vi "2DRasterScanWithScopeCommAndSafeRetract.vi"() -> ()   [LabVIEW 2015]
panel:
  in  "Swap X and Z?":bool
  out "Progress":u8(slide)=96 scale=0.0..100.0
  out "Z-error":errorcluster
  out "X-error":errorcluster
  in  "Z safe retract":sgl=25.0
  in  "MG17Motor Z axis":refnum<k7>(container)
  in  "Home Z?":bool
  in  "Z-Axis Serial":i32=27001113
  in  "Safe retract?":bool=TRUE
  in  "X safe retract":sgl=100.0
  in  "Y safe retract":sgl=25.0
  out "Y error":errorcluster
  in  "Base filename":string="TDS" caption="Filename"
  in  "Save Each Point":bool=TRUE
  in  "X-Axis Serial":i32=45869591
  in  "Y-Axis Serial":i32=27501169
  out "Number of movements for Y stage":sgl=49.0
  in  "Distance from center X axis (mm)":dbl=2.0 step=0.001
  in  "Movement Step Size X axis (mm)":sgl=0.25 step=0.001
  in  "Channel Select":T1(ring)=enum."Channel 1"
  in  "Selected Directory":path=path "C:/Users/admin.WIN10DC20170225/Documents/Hydrophone Data/TDS Scans/TDS 04_04_18 BarePZT-20ms-XY"
  in  "Stage Max Velocity (mm/s)":sgl=1.5
  in  "Stage Acceleration (mm/s²)":sgl=1.0
  in  "Stage Minimum Velocity (mm/s)":sgl
  in  "Center point Y axis (mm)":dbl=20.0 step=0.001 format="%#_13g"
  in  "Center point X axis (mm)":dbl=63.5 step=0.001 format="%#_13g"
  out "Number of movements for X stage":sgl=49.0
  in  "Distance from center Y axis (mm)":dbl=2.0 step=0.001
  in  "MG17Motor X axis":refnum<k7>(container)
  in  "Home stages\nbefore scanning":bool caption="Do this each time LabVIEW  is opened, controllers are unplugged, or stages are disconnected."
  in  "error in (no error)":errorcluster
  in  "MG17Motor Y axis":refnum<k7>(container)
  out "Current position in line":i32=49
  out "Current line number":i32=49
  in  "Movement Step Size Y axis (mm)":sgl=0.25 step=0.001
  # "BEFORE STARTING SCAN ENSURE THAT X-Z AXIS SWAPPING AND SAFE RETRACT VALUES ARE PROPERLY SET"
  # "Use safe retract to pull hydrophone out of water when scan is finished. Normal retraction order is Y -> X -> Z"
  # "When X and Z are swapped,\nretraction order is Y -> Z -> X"
  # "For Y-Z scans- turn this on and then treat X values as Z."
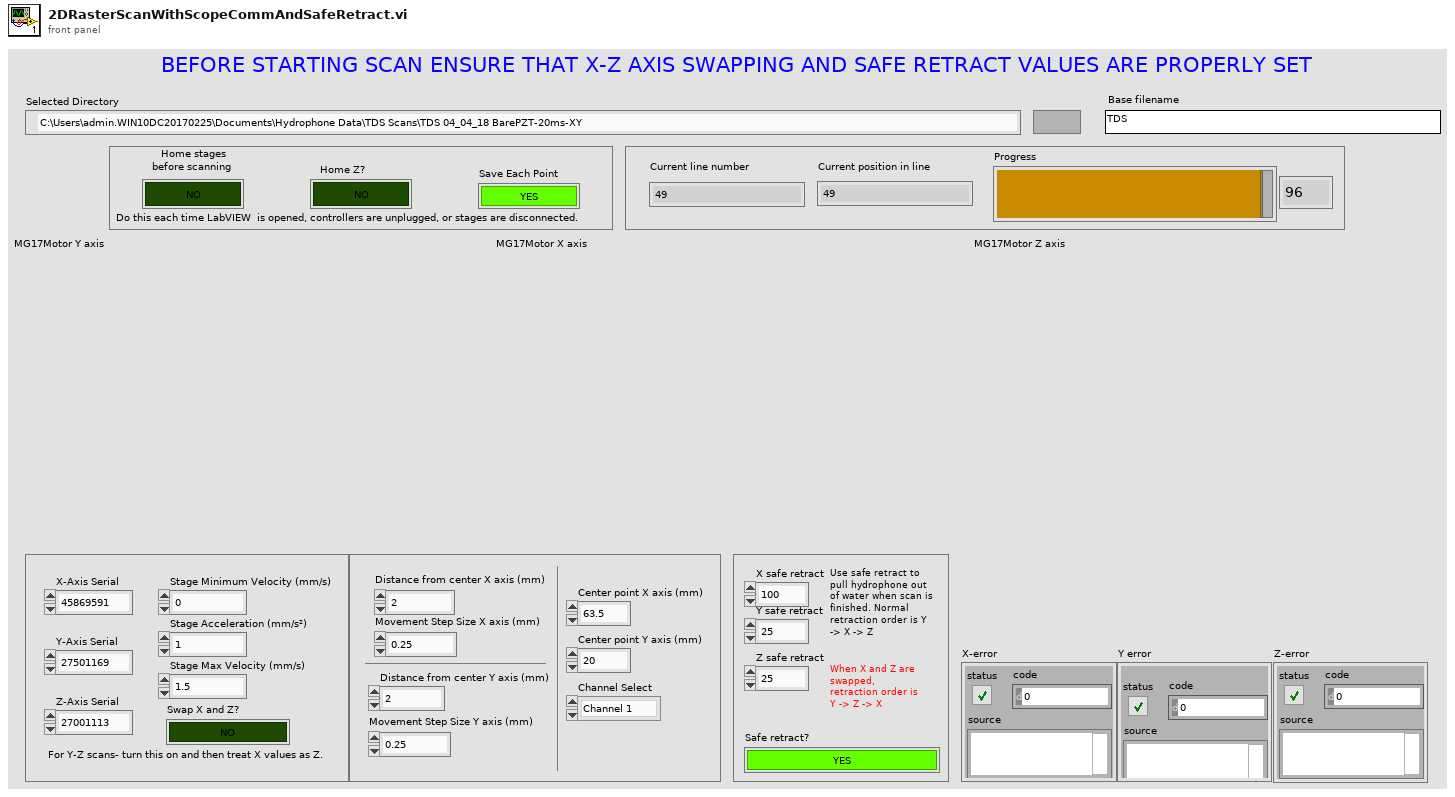
[diagram p1: front panel]
types:
  T1 = enum16{"Trace D", "Trace C", "Trace B", "Trace A", "Channel 4", "Channel 3", "Channel 2", "Channel 1"}
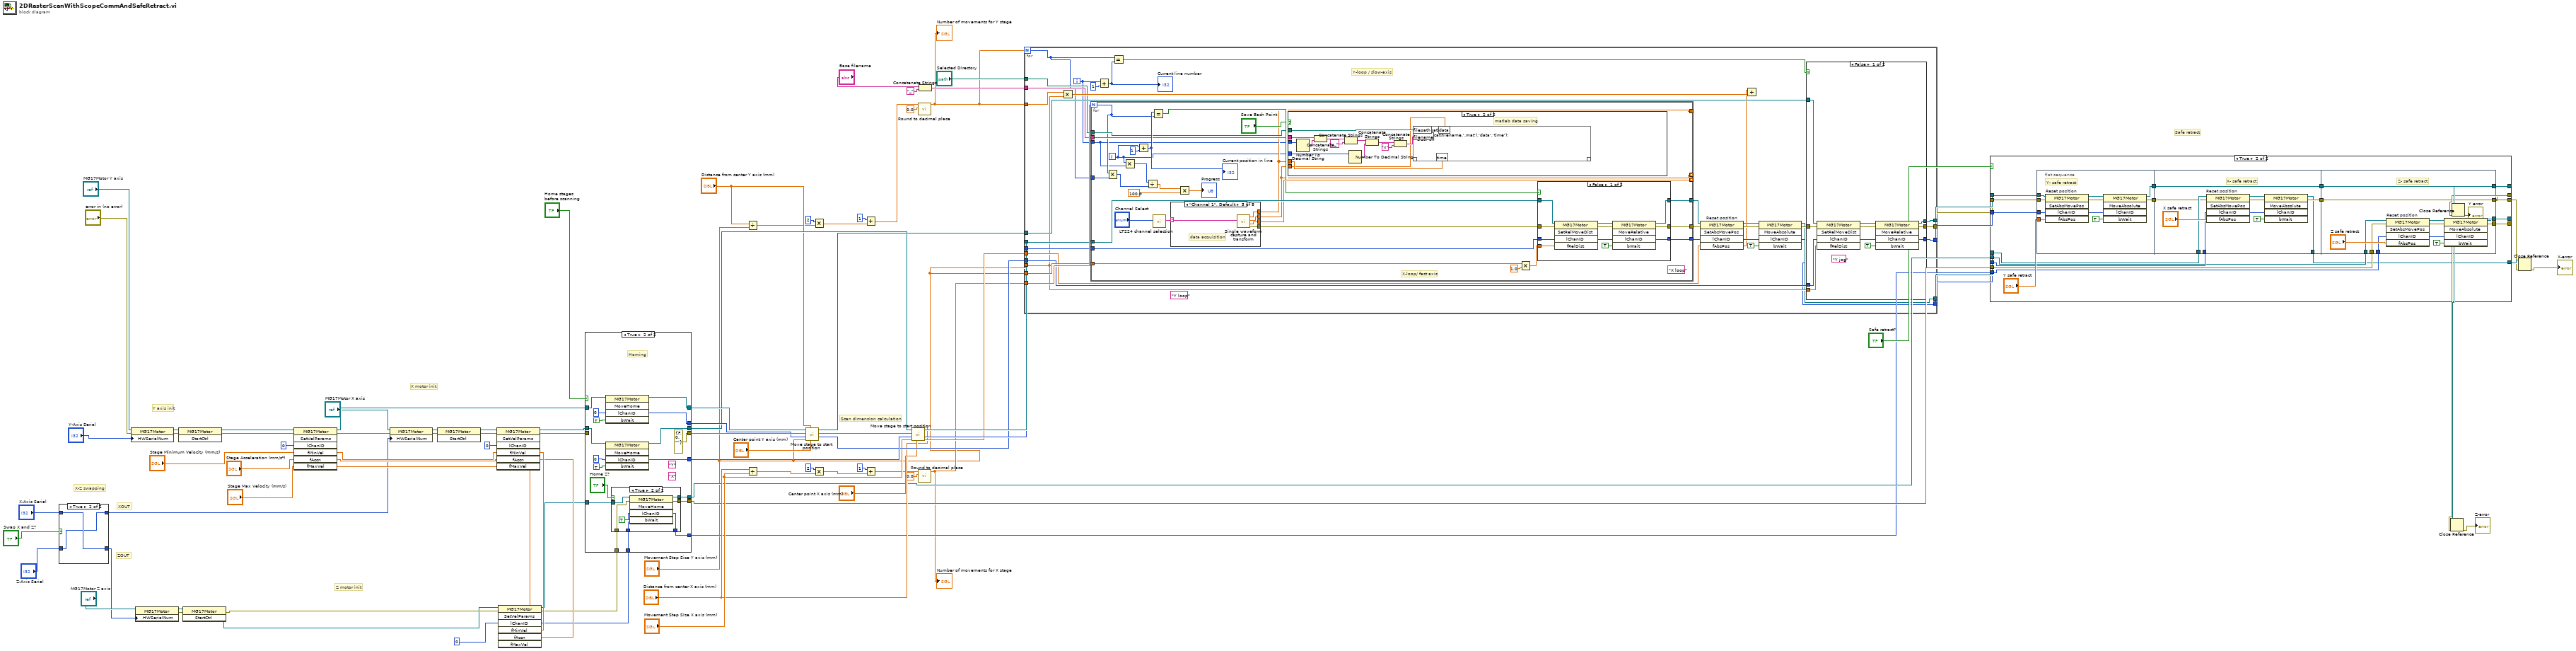
[diagram p0: block diagram]
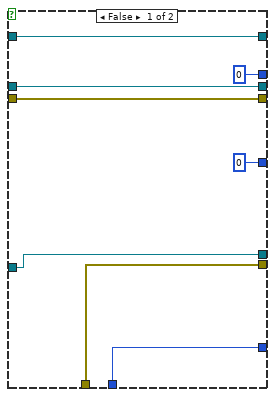
[diagram p4: hidden frame]
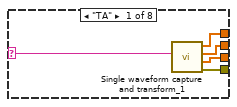
[diagram p9: hidden frame]
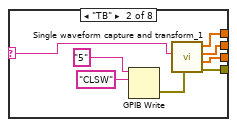
[diagram p10: hidden frame]
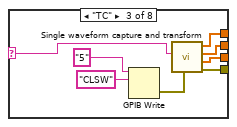
[diagram p11: hidden frame]
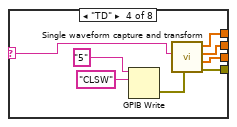
[diagram p12: hidden frame]
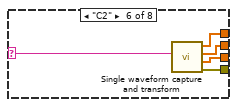
[diagram p13: hidden frame]
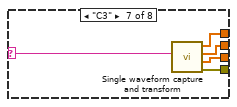
[diagram p14: hidden frame]
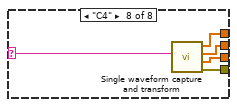
[diagram p15: hidden frame]
diagram:
  # "Scan dimension calculation"
  # "X-Z swapping"
  # "Y axis init"
  # "Z motor init"
  # "X motor init"
  # "ZOUT"
  # "XOUT"
  # "Safe retract"
  n1 = case shown="True" "Swap X and Z?" {
    tunnel: "X-Axis Serial" -> [w97 w99]
    tunnel: [w97 w98] -> w6
    tunnel: "Z-Axis Serial" -> [w96 w98]
    tunnel: [w96 w99] -> w5
    frame False {
    }
    frame True {
    }
  }
  n2 = property on="Property Node" class="MG17Motor"(reference="MG17Motor Y axis", error in="error in (no error)", "HWSerialNum"="Y-Axis Serial") -> (reference out=w94:refnum<k7>, error out=w93:errorcluster)
  n3 = property on="Property Node" class="MG17Motor"(reference="MG17Motor Z axis", "HWSerialNum"=w5) -> (reference out=w27:refnum<k7>, error out=w28:errorcluster)  [unwired: 1 in]
  n4 = invoke class="MG17Motor" method="StartCtrl"(reference=w94, error in=w93) -> (reference out=w86:refnum<k7>, error out=w87:errorcluster)  [unwired: 1 in, 1 out]
  n5 = invoke class="MG17Motor" method="StartCtrl"(reference=w27, error in=w28) -> (reference out=w23:refnum<k7>, error out=w22:errorcluster)  [unwired: 1 in, 1 out]
  n6 = invoke class="MG17Motor" method="SetVelParams"(reference=w86, error in=w87, "lChanID"=0, "fMinVel"="Stage Minimum Velocity (mm/s)", "fAccn"="Stage Acceleration (mm/s²)", "fMaxVel"="Stage Max Velocity (mm/s)") -> (reference out=w75:refnum<k7>, error out=w76:errorcluster, "fMinVel"=w56:sgl, "fAccn"=w55:sgl, "fMaxVel"=w54:sgl)  [unwired: 1 in, 2 out]
  n7 = property on="Property Node" class="MG17Motor"(reference="MG17Motor X axis", error in=w76, "HWSerialNum"=w6) -> (reference out=w89:refnum<k7>, error out=w88:errorcluster)
  n8 = invoke class="MG17Motor" method="StartCtrl"(reference=w89, error in=w88) -> (reference out=w85:refnum<k7>, error out=w78:errorcluster)  [unwired: 1 in, 1 out]
  n9 = invoke class="MG17Motor" method="SetVelParams"(reference=w85, error in=w78, "lChanID"=0, "fMinVel"=w56, "fAccn"=w55, "fMaxVel"=w54) -> (reference out=w84:refnum<k7>, error out=w77:errorcluster, "fMinVel"=w26:sgl, "fAccn"=w25:sgl, "fMaxVel"=w24:sgl)  [unwired: 1 in, 2 out]
  n10 = invoke class="MG17Motor" method="SetVelParams"(reference=w23, error in=w22, "lChanID"=0, "fMinVel"=w26, "fAccn"=w25, "fMaxVel"=w24) -> (reference out=w20:refnum<k7>, error out=w19:errorcluster, "lChanID"=w14:i32)  [unwired: 1 in, 4 out]
  n11 = case shown="True" "Home stages\nbefore scanning" {
    tunnel: [w104 w121] -> w65
    tunnel: [w105 w120] -> w71
    tunnel: [0 ("lChanID") w119] -> w66
    tunnel: [0 ("lChanID") w118] -> w69
    tunnel: [w103 errorcluster {"status"=FALSE, "code"=0, "source"=""} ("error out")] -> w70
    tunnel: w75 -> [w105 w116]
    tunnel: w84 -> [w104 w115]
    tunnel: w77 -> [w103 _]
    tunnel: w20 -> [w102 w113]
    tunnel: w19 -> [w101 w112]
    tunnel: [w102 w111] -> w17
    tunnel: [w101 w110] -> w16
    tunnel: w14 -> [w100 w109]
    tunnel: [w100 w108] -> w13
    frame False {
    }
    frame True {
      (unwired) "X"
      (unwired) "Y"
      # "Homing"
      n12 = invoke class="MG17Motor" method="MoveHome"(reference=w116, "lChanID"=0, "bWait"=TRUE) -> (reference out=w120:refnum<k7>, "lChanID"=w118:i32)  [unwired: 2 in, 3 out]
      n13 = invoke class="MG17Motor" method="MoveHome"(reference=w115, "lChanID"=0, "bWait"=TRUE) -> (reference out=w121:refnum<k7>, "lChanID"=w119:i32)  [unwired: 2 in, 3 out]
      n14 = case shown="True" "Home Z?" {
        tunnel: w113 -> [w128 w134]
        tunnel: w112 -> [w127 w133]
        tunnel: [w128 w132] -> w111
        tunnel: [w127 w131] -> w110
        tunnel: w109 -> [w126 w130]
        tunnel: [w126 w129] -> w108
        frame False {
        }
        frame True {
          n15 = invoke class="MG17Motor" method="MoveHome"(reference=w134, error in=w133, "lChanID"=w130, "bWait"=TRUE) -> (reference out=w132:refnum<k7>, error out=w131:errorcluster, "lChanID"=w129:i32)  [unwired: 1 in, 2 out]
        }
      }
    }
  }
  n16 = Divide(x="Distance from center Y axis (mm)", y="Movement Step Size Y axis (mm)") -> (x/y=w59:dbl)
  n17 = Divide(x="Distance from center X axis (mm)", y="Movement Step Size X axis (mm)") -> (x/y=w51:dbl)
  n18 = call "Move stage to start position.vi"("Center point of axis (mm)"="Center point Y axis (mm)", "Distance from center (mm)"="Distance from center Y axis (mm)", "Movement Step Size (mm)"="Movement Step Size Y axis (mm)", "lChanID"=w69, "error in"=w70, "reference in"=w71) -> ("lChanID out"=w60:i32, "error out"=w67:errorcluster, "reference out"=w68:refnum<k7>)  [unwired: 2 in, 1 out]
  n19 = Multiply(x=2, y=w59) -> (x*y=w73:dbl)
  n20 = Multiply(x=2, y=w51) -> (x*y=w52:dbl)
  n21 = Add(x=1, y=w73) -> (x+y=w46:dbl)
  n22 = Add(x=1, y=w52) -> (x+y=w47:dbl)
  n23 = call "Move stage to start position.vi"("Center point of axis (mm)"="Center point X axis (mm)", "Distance from center (mm)"="Distance from center X axis (mm)", "Movement Step Size (mm)"="Movement Step Size X axis (mm)", "lChanID"=w66, "error in"=w67, "reference in"=w65) -> ("Start position out"=w61:sgl, "lChanID out"=w62:i32, "reference out"=w63:refnum<k7>)  [unwired: 2 in, 1 out]
  n24 = call "Round to decimal place.vi"("Power of ten"=0.0, "Number to round"=w46) -> ("Rounded number"=w1:dbl)  [unwired: 8 in, 1 out]
  "Number of movements for Y stage" <- w1
  n25 = call "Round to decimal place.vi"("Power of ten"=0.0, "Number to round"=w47) -> ("Rounded number"=w4:dbl)  [unwired: 8 in, 1 out]
  "Number of movements for X stage" <- w4
  n26 = Concatenate Strings("Base filename", "_" ("string")) -> (w40:string)
  n27 = for {
    N: w1 -> [w137]
    tunnel: "Movement Step Size Y axis (mm)" -> [w161]
    tunnel: w4 -> [w166]
    tunnel: [w156] -> w37
    tunnel: [w155] -> w12
    tunnel: "Movement Step Size Y axis (mm)" -> [w148]
    tunnel: w68 -> [w154]
    tunnel: w63 -> [w153]
    tunnel: w62 -> [w152]
    tunnel: w61 -> [w151]
    tunnel: w60 -> [w150]
    tunnel: w1 -> [w147]
    tunnel: w40 -> [w143]
    tunnel: "Selected Directory" -> [w142]
    tunnel: [w140] -> w35
    tunnel: [w139] -> w36
    tunnel: [w138] -> w34
    i -> [w141]
    (unwired) "Y loop"
    # "Y-loop / slow-axis"
    n28 = Multiply(x=w147, y=w148) -> (x*y=w149:dbl)
    n29 = for {
      N: w166 -> [w188]
      tunnel: w161 -> [w201]
      tunnel: [w190] -> _
      tunnel: [w205] -> w144
      tunnel: [w206] -> w159
      tunnel: [w204] -> w158
      tunnel: [w198] -> _ mode=indexing
      tunnel: w153 -> [w202]
      tunnel: w152 -> [w203]
      tunnel: [w193] -> _ mode=indexing
      tunnel: w143 -> [w194]
      tunnel: w142 -> [w192]
      tunnel: w141 -> [w187]
      tunnel: w137 -> [w189]
      i -> [w184]
      (unwired) "X loop"
      # "X-loop/ fast axis"
      n30 = Multiply(x=w188, y=w189) -> (x*y=w181:i32)
      n31 = Multiply(x=w184, y=w187) -> (x*y=w182:i32)
      n32 = Add(x=w184, y=1) -> (x+y=w195:i32)
      "Current position in line" <- w195
      n33 = Divide(x=w182, y=w181) -> (x/y=w183:dbl)
      n34 = Equal?(x=w195, y=w188) -> (x = y?=w196:bool)
      n35 = call "LT224 channel selection.vi"("Channel Select"="Channel Select") -> ("Selected channel"=w199:string)  [unwired: 10 in]
      n36 = case shown="\"Channel 1\", Default" w199 {
        selector: w199 -> [w239 w244 w252 w260 w268 w273 w278 w283]
        tunnel: [w242 w250 w258 w266 w271 w276 w281 w286] -> w197
        tunnel: [w241 w249 w257 w265 w270 w275 w280 w285] -> w198
        tunnel: [w240 w248 w256 w264 w269 w274 w279 w284] -> w190
        tunnel: [w238 w243 w251 w259 w267 w272 w277 w282] -> w193
        frame "TA" {
          n37 = call "Single waveform capture and transform_1.vi"("channel name (\"\")"=w239) -> ("error out"=w242:errorcluster, "Transformed waveform vector"=w241:dbl[], "waveform vector"=w238:dbl[], "Time vector"=w240:dbl[])  [unwired: 7 in]
        }
        frame "TB" {
          n38 = GPIB Write(0:"5" ("address string"), 1:"CLSW" ("data")) -> (6:w246:errorcluster)  [unwired: 3 in, 1 out]
          n39 = call "Single waveform capture and transform_1.vi"("error in"=w246, "channel name (\"\")"=w244) -> ("error out"=w250:errorcluster, "Transformed waveform vector"=w249:dbl[], "waveform vector"=w243:dbl[], "Time vector"=w248:dbl[])  [unwired: 6 in]
        }
        frame "TC" {
          n40 = GPIB Write(0:"5" ("address string"), 1:"CLSW" ("data")) -> (6:w254:errorcluster)  [unwired: 3 in, 1 out]
          n41 = call "Single waveform capture and transform.vi"("error in"=w254, "channel name (\"\")"=w252) -> ("error out"=w258:errorcluster, "Transformed waveform vector"=w257:dbl[], "waveform vector"=w251:dbl[], "Time vector"=w256:dbl[])  [unwired: 6 in]
        }
        frame "TD" {
          n42 = GPIB Write(0:"5" ("address string"), 1:"CLSW" ("data")) -> (6:w262:errorcluster)  [unwired: 3 in, 1 out]
          n43 = call "Single waveform capture and transform.vi"("error in"=w262, "channel name (\"\")"=w260) -> ("error out"=w266:errorcluster, "Transformed waveform vector"=w265:dbl[], "waveform vector"=w259:dbl[], "Time vector"=w264:dbl[])  [unwired: 6 in]
        }
        frame "Channel 1", Default {
          # "data acquisition"
          n44 = call "Single waveform capture and transform.vi"("channel name (\"\")"=w268) -> ("error out"=w271:errorcluster, "Transformed waveform vector"=w270:dbl[], "waveform vector"=w267:dbl[], "Time vector"=w269:dbl[])  [unwired: 7 in]
        }
        frame "C2" {
          n45 = call "Single waveform capture and transform.vi"("channel name (\"\")"=w273) -> ("error out"=w276:errorcluster, "Transformed waveform vector"=w275:dbl[], "waveform vector"=w272:dbl[], "Time vector"=w274:dbl[])  [unwired: 7 in]
        }
        frame "C3" {
          n46 = call "Single waveform capture and transform.vi"("channel name (\"\")"=w278) -> ("error out"=w281:errorcluster, "Transformed waveform vector"=w280:dbl[], "waveform vector"=w277:dbl[], "Time vector"=w279:dbl[])  [unwired: 7 in]
        }
        frame "C4" {
          n47 = call "Single waveform capture and transform.vi"("channel name (\"\")"=w283) -> ("error out"=w286:errorcluster, "Transformed waveform vector"=w285:dbl[], "waveform vector"=w282:dbl[], "Time vector"=w284:dbl[])  [unwired: 7 in]
        }
      }
      n48 = Multiply(x=w183, y=100.0) -> (x*y=→"Progress":dbl)
      n49 = case shown="True" "Save Each Point" {
        tunnel: w194 -> [_ w215]
        tunnel: w193 -> [_ w210]
        tunnel: w192 -> [_ w213]
        tunnel: w184 -> [_ w223]
        tunnel: w187 -> [_ w217]
        tunnel: w190 -> [_ w211]
        frame False {
        }
        frame True {
          # "matlab data saving"
          n50 = Number To Decimal String(number=w217) -> (decimal integer string=w214:string)  [unwired: 1 in]
          n51 = Concatenate Strings(w215, w214) -> (w222:string)
          n52 = Concatenate Strings(w222, "y_" ("string")) -> (w220:string)
          n53 = Number To Decimal String(number=w223) -> (decimal integer string=w216:string)  [unwired: 1 in]
          n54 = Concatenate Strings(w220, w216) -> (w218:string)
          n55 = Concatenate Strings(w218, "x" ("string")) -> (w212:string)
          n56 = script code="cd(filepath)\nsave(strcat(filename,'.mat'),'data','time');\nclear all"("filename"=w212, "filepath"=w213, "time"=w211, "data"=w210) -> ()  [unwired: 1 in, 1 out]
        }
      }
      n57 = Multiply(x=w201, y=sgl 1.0) -> (x*y=w208:sgl)
      n58 = case shown="False" w196 {
        tunnel: w208 -> [w234 _]
        tunnel: [w229 w235] -> w206
        tunnel: [w228 w237] -> w205
        tunnel: [w227 w236] -> w204
        tunnel: w203 -> [w226 w236]
        tunnel: w202 -> [w225 w235]
        tunnel: w197 -> [w224 w237]
        frame False {
          n59 = invoke class="MG17Motor" method="SetRelMoveDist"(reference=w225, error in=w224, "lChanID"=w226, "fRelDist"=w234) -> (reference out=w232:refnum<k7>, error out=w231:errorcluster, "lChanID"=w233:i32)  [unwired: 1 in, 2 out]
          n60 = invoke class="MG17Motor" method="MoveRelative"(reference=w232, error in=w231, "lChanID"=w233, "bWait"=TRUE) -> (reference out=w229:refnum<k7>, error out=w228:errorcluster, "lChanID"=w227:i32)  [unwired: 1 in, 2 out]
        }
        frame True {
        }
      }
    }
    n61 = Add(x=w141, y=1) -> (x+y=w145:i32)
    "Current line number" <- w145
    n62 = Equal?(x=w137, y=w145) -> (x = y?=w136:bool)
    n63 = invoke on="Reset position" class="MG17Motor" method="SetAbsMovePos"(reference=w159, error in=w144, "lChanID"=w158, "fAbsPos"=w151) -> (reference out=w162:refnum<k7>, error out=w164:errorcluster, "lChanID"=w163:i32, "fAbsPos"=w146:sgl)  [unwired: 1 in, 1 out]
    n64 = Add(x=w146, y=w149) -> ()  [unwired: 1 out]
    n65 = invoke class="MG17Motor" method="MoveAbsolute"(reference=w162, error in=w164, "lChanID"=w163, "bWait"=TRUE) -> (reference out=w139:refnum<k7>, error out=w157:errorcluster, "lChanID"=w138:i32)  [unwired: 1 in, 2 out]
    n66 = case shown="False" w136 {
      tunnel: w157 -> [w173 w180]
      tunnel: [w172 w178] -> w156
      tunnel: [w171 w180] -> w140
      tunnel: [w170 w179] -> w155
      tunnel: w148 -> [w169 _]
      tunnel: w154 -> [w168 w178]
      tunnel: w150 -> [w167 w179]
      frame False {
        (unwired) "Y jog"
        n67 = invoke class="MG17Motor" method="SetRelMoveDist"(reference=w168, error in=w173, "lChanID"=w167, "fRelDist"=w169) -> (reference out=w175:refnum<k7>, error out=w176:errorcluster, "lChanID"=w174:i32)  [unwired: 1 in, 2 out]
        n68 = invoke class="MG17Motor" method="MoveRelative"(reference=w175, error in=w176, "lChanID"=w174, "bWait"=TRUE) -> (reference out=w172:refnum<k7>, error out=w171:errorcluster, "lChanID"=w170:i32)  [unwired: 1 in, 2 out]
      }
      frame True {
      }
    }
  }
  n69 = case shown="True" "Safe retract?" {
    tunnel: w37 -> [w291 w309]
    tunnel: w36 -> [w290 w303]
    tunnel: w35 -> [w289 w307]
    tunnel: w34 -> [_ w301]
    tunnel: [w291 w306] -> w33
    tunnel: [w289 w292] -> w32
    tunnel: [w290 w293] -> w31
    tunnel: [w289 w292] -> w30
    tunnel: w17 -> [w288 w297]
    tunnel: w16 -> [w287 w296]
    tunnel: [w288 w298] -> w15
    tunnel: [w287 w294] -> w2
    tunnel: w13 -> [_ w295]
    tunnel: w12 -> [_ w302]
    frame False {
    }
    frame True {
      n70 = flat-sequence {
        tunnel: w309 -> [w315]
        tunnel: "Y safe retract" -> [w314]
        tunnel: w307 -> [w313]
        tunnel: [w312] -> w305
        tunnel: [w311] -> w304
        tunnel: w302 -> [w310]
        tunnel: w305 -> [w323]
        tunnel: w304 -> [w322]
        tunnel: w303 -> [w325]
        tunnel: w301 -> [w324]
        tunnel: [w323] -> w300
        tunnel: [w321] -> w299
        tunnel: [w320] -> w293
        tunnel: [w331] -> w292
        tunnel: [w342] -> w306
        tunnel: w300 -> [w342]
        tunnel: w299 -> [w331]
        tunnel: [w336] -> w298
        tunnel: w297 -> [w335]
        tunnel: w296 -> [w334]
        tunnel: w295 -> [w333]
        tunnel: [w332] -> w294
        frame #0 {
          # "Y- safe retract"
          n71 = invoke on="Reset position" class="MG17Motor" method="SetAbsMovePos"(reference=w315, error in=w313, "lChanID"=w310, "fAbsPos"=w314) -> (reference out=w319:refnum<k7>, error out=w318:errorcluster, "lChanID"=w317:i32)  [unwired: 1 in, 2 out]
          n72 = invoke class="MG17Motor" method="MoveAbsolute"(reference=w319, error in=w318, "lChanID"=w317, "bWait"=TRUE) -> (reference out=w312:refnum<k7>, error out=w311:errorcluster)  [unwired: 1 in, 3 out]
        }
        frame #1 {
          # "X- safe retract"
          n73 = invoke on="Reset position" class="MG17Motor" method="SetAbsMovePos"(reference=w325, error in=w322, "lChanID"=w324, "fAbsPos"="X safe retract") -> (reference out=w326:refnum<k7>, error out=w327:errorcluster, "lChanID"=w330:i32)  [unwired: 1 in, 2 out]
          n74 = invoke class="MG17Motor" method="MoveAbsolute"(reference=w326, error in=w327, "lChanID"=w330, "bWait"=TRUE) -> (reference out=w320:refnum<k7>, error out=w321:errorcluster)  [unwired: 1 in, 3 out]
        }
        frame #2 {
          # "Z- safe retract"
          n75 = invoke on="Reset position" class="MG17Motor" method="SetAbsMovePos"(reference=w335, error in=w334, "lChanID"=w333, "fAbsPos"="Z safe retract") -> (reference out=w337:refnum<k7>, error out=w338:errorcluster, "lChanID"=w339:i32)  [unwired: 1 in, 2 out]
          n76 = invoke class="MG17Motor" method="MoveAbsolute"(reference=w337, error in=w338, "lChanID"=w339, "bWait"=TRUE) -> (reference out=w336:refnum<k7>, error out=w332:errorcluster)  [unwired: 1 in, 3 out]
        }
      }
    }
  }
  n77 = Close Reference(reference=w15, error in (no error)=w2) -> (error out=→"Z-error":errorcluster)
  n78 = Close Reference(reference=w33, error in (no error)=w32) -> (error out=→"Y error":errorcluster)
  n79 = Close Reference(reference=w31, error in (no error)=w30) -> (error out=→"X-error":errorcluster)
